vi "Log_B.vi"(1 "Data":string, 2 "number of bytes in buffer_data":i32, 12 "error in (no error)":errorcluster) -> (3 "Data dup":string, 14 "error out":errorcluster)   [LabVIEW 2014]
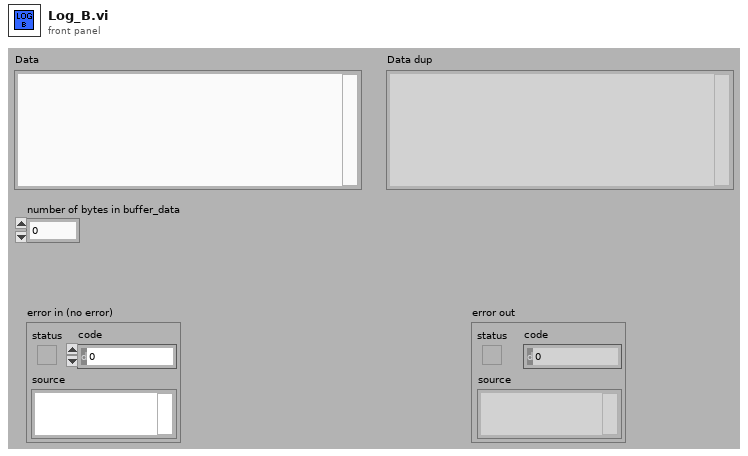
[diagram p1: front panel]
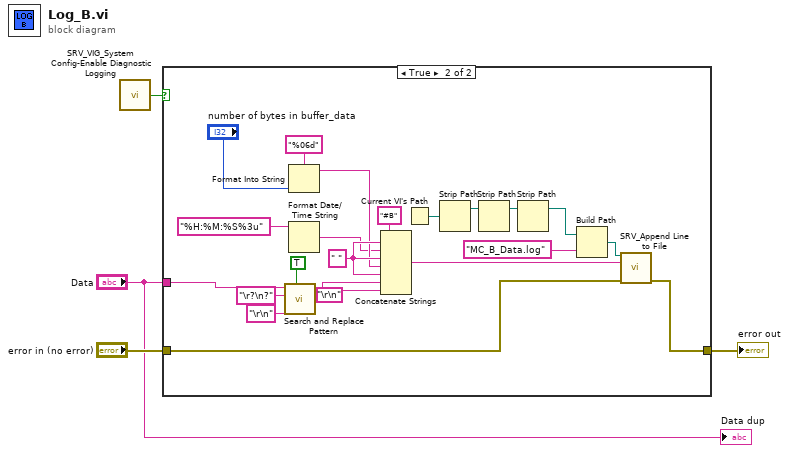
[diagram p0: block diagram]
diagram:
  n1 = call "SRV_VIG_System Config-Enable Diagnostic Logging.vi"() -> ("Enable Diagnostic Log?"=w1:bool)  [unwired: 15 in]
  n2 = case shown="True" w1 {
    tunnel: [w5 w25] -> w4
    tunnel: "error in (no error)" -> [w5 w24]
    tunnel: "Data" -> [_ w7]
    frame False {
    }
    frame True {
      w15 = " " ("string")
      n3 = call <vilib>:"Search and Replace Pattern.vi"("string"=w7, "regular expression (\"\")"="\r?\n?" ("regular expression (\"\")"), "replace string (\"\")"="\r\n" ("replace string (\"\")"), "replace all? (F)"=TRUE) -> ("result string"=w6:string)  [unwired: 1 in, 1 out]
      n4 = Format Into String(format string="%06d", "number of bytes in buffer_data") -> (resulting string=w13:string)  [unwired: 2 in, 1 out]
      n5 = Format Date/Time String(time format string (%c)="%H:%M:%S%3u") -> (date/time string=w12:string)  [unwired: 2 in]
      n6 = Concatenate Strings("#B" ("string"), w15, w12, w15, w13, w15, w6, "\r\n") -> (w26:string)
      n7 = Current VI's Path() -> (path=w19:path)
      n8 = Strip Path(path=w19) -> (stripped path=w20:path)  [unwired: 1 out]
      n9 = Strip Path(path=w20) -> (stripped path=w21:path)  [unwired: 1 out]
      n10 = Strip Path(path=w21) -> (stripped path=w18:path)  [unwired: 1 out]
      n11 = Build Path(base path=w18, name or relative path="MC_B_Data.log") -> (appended path=w22:path)
      n12 = call "SRV_Append Line to File.vi"("file path"=w22, "Line to Write"=w26, "error in (no error)"=w24) -> ("error out"=w25:errorcluster)  [unwired: 12 in]
    }
  }
  "error out" <- w4
  "Data dup" <- "Data"
